vi "Property Dialog_Toggle RW Symbol.vi"(5 "Prior Property Array":T1(array[cluster]), 6 "Shift click?":bool, 7 "Action":T2, 8 "Error In":errorcluster, 9 "Coords":cluster{"Horizontal":i32, "Vertical":i32}, 10 "Tree Control in":refnum<vi>, 11 "All Tree Refs":refnum<vi>[](array[refnum])) -> (0 "Error Out":errorcluster, 1 "Tag Selected":string[](array[string]), 2 "Tree Control Out":refnum<vi>)   [LabVIEW 2023]
uses:
  controls/action enum.ctl
panel:
  out "subarray":string[](array[string])
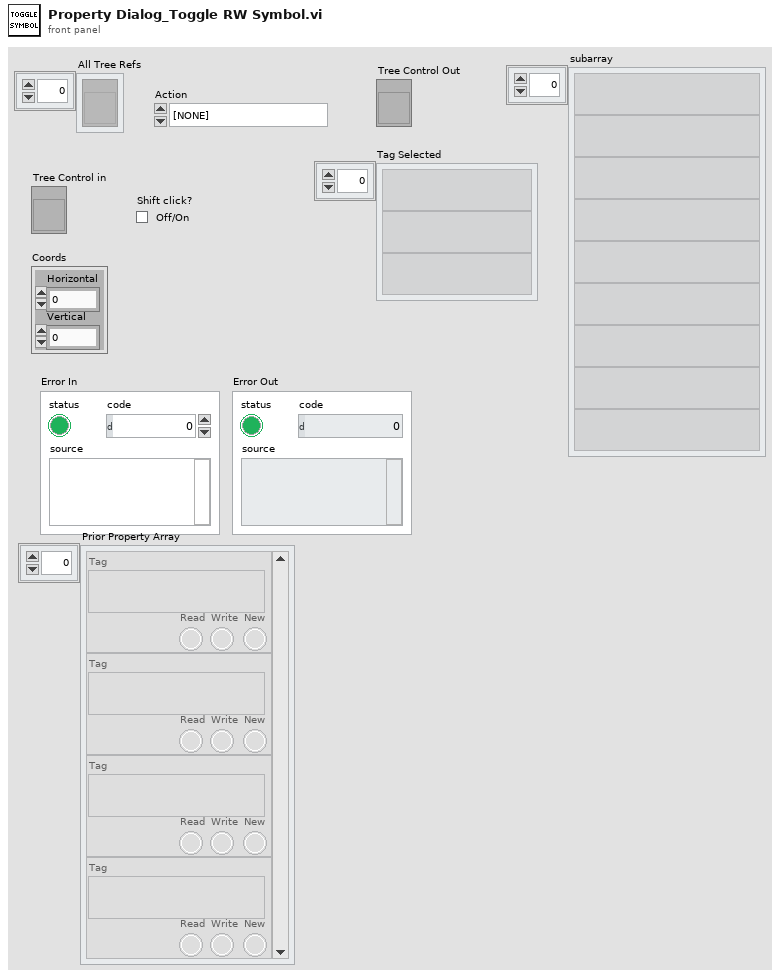
[diagram p1: front panel]
types:
  T1 = cluster{"Tag":string, "Read":bool, "Write":bool, "New":bool}[]
  T2 = typedef "action enum.ctl" = enum16{"[NONE]", "Wire Bundle", "Wire Unbundle", "Terminal Unbundle", "Terminal Bundle", "Bundler Move Up", "Bundler Move Down", "Bundler Insert", "Bundler Remove", "Bundler Remove Unwired", "Bundler Rearrange", "In Place Insert", "In Place Remove", "In Place Remove Unwired", "In Place Rearrange", "Wire Properties", "Wire Method", "Terminal Properties", "Terminal Method", "Property Move Up", "Property Move Down", "Properties Insert", "Properties Remove", "Properties Remove Unwired", "Properties Rearrange", "Method Change", "Class for Constant", "Class For Control", "Class For Node", "Class Name to Clipboard"}
  T3 = enum16{"Init", "Read", "Remove", "Remove or Append", "Append", "Append If New"}
  T4 = cluster{"Tag":string, "Read":bool, "Write":bool, "New":bool}
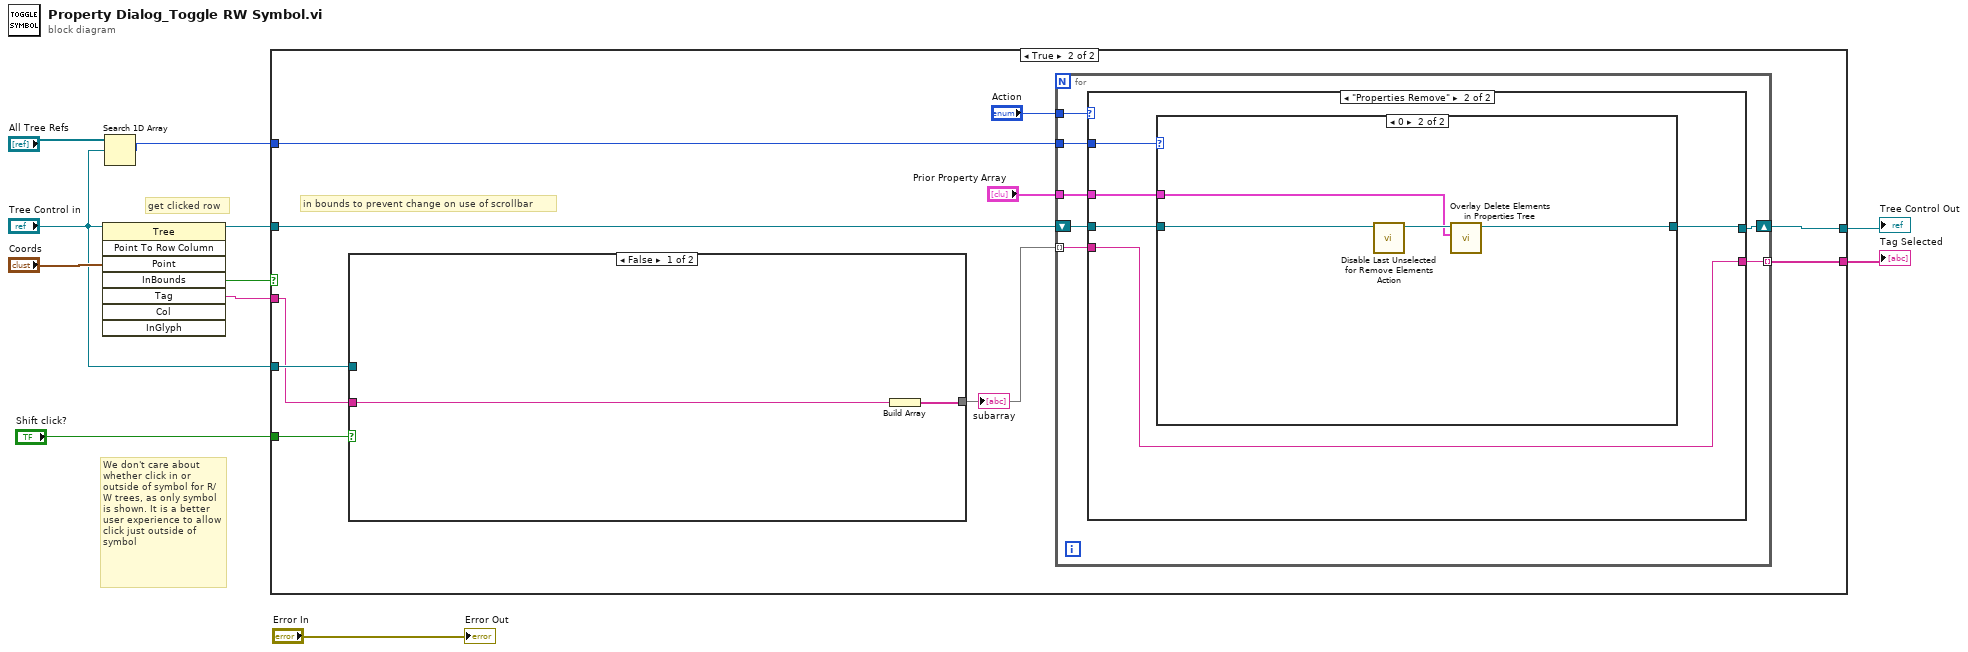
[diagram p0: block diagram]
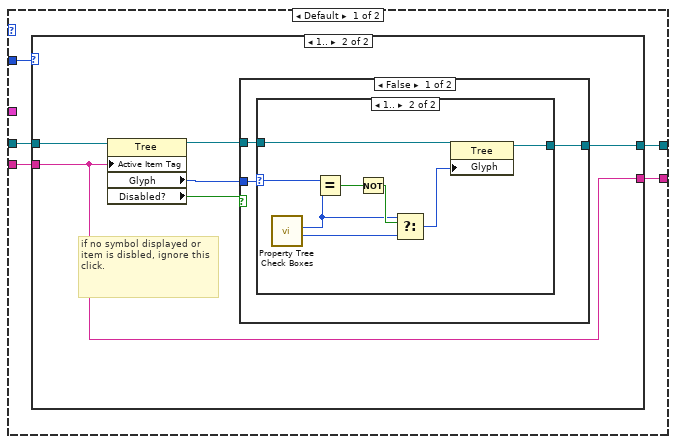
[diagram p3: hidden frame]
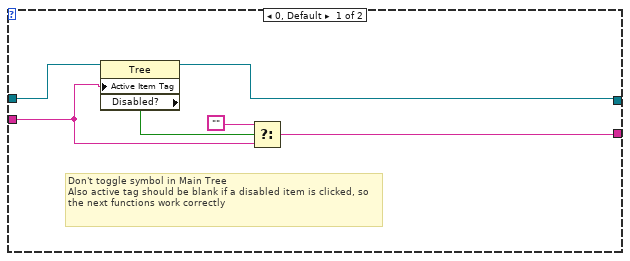
[diagram p4: hidden frame]
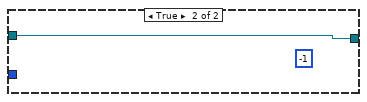
[diagram p6: hidden frame]
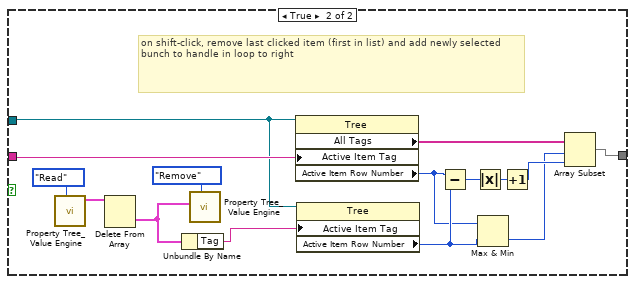
[diagram p8: hidden frame]
diagram:
  # "We don't care about whether click in or outside of symbol for R/W trees, as only symbol is shown. It is a better user experience to allow click just outside of symbol"
  # "get clicked row"
  n1 = invoke class="Tree" method="Point To Row Column"(reference="Tree Control in", "Point"="Coords") -> (reference out=w10:refnum<vi>, "InBounds"=w2:bool, "Tag"=w5:string)  [unwired: 6 in, 5 out]
  n2 = Search 1D Array(1D array="All Tree Refs", element="Tree Control in") -> (index of element=w8:i32)  [unwired: 1 in]
  n3 = case shown="True" w2 {
    tunnel: w10 -> [_ w21]
    tunnel: w8 -> [_ w20]
    tunnel: "Shift click?" -> [_ w18]
    tunnel: "Tree Control in" -> [_ w17]
    tunnel: w5 -> [_ w16]
    tunnel: [_ w14] -> w4
    tunnel: [_ w13] -> w3
    frame False {
    }
    frame True {
      # "in bounds to prevent change on use of scrollbar"
      n4 = case shown="False" w18 {
        tunnel: w17 -> [_ w73]
        tunnel: w16 -> [w70 w75]
        tunnel: [w69 w74] -> w15
        frame False {
          n5 = Build Array(w70) -> (w69:string[])
        }
        frame True {
          # "on shift-click, remove last clicked item (first in list) and add newly selected bunch to handle in loop to right"
          n6 = call "Property Tree_Value Engine.vi"("Save Action"=T3."Read" ("Action")) -> ("Property Array Out"=w85:T1)  [unwired: 8 in, 2 out]
          n7 = Delete From Array(array=w85) -> (deleted portion=w84:T4)  [unwired: 2 in, 1 out]
          n8 = Unbundle By Name(w84) -> ("Tag"=w76:string)
          n9 = call "Property Tree_Value Engine.vi"("Save Action"=T3."Remove" ("Action"), "Element"=w84) -> ()  [unwired: 7 in, 3 out]
          n10 = property class="Tree"(reference=w73, "Active Item Tag"=w75) -> ("All Tags"=w78:string[], "Active Item Row Number"=w79:i32)  [unwired: 1 in, 2 out]
          n11 = property class="Tree"(reference=w73, "Active Item Tag"=w76) -> ("Active Item Row Number"=w80:i32)  [unwired: 1 in, 2 out]
          n12 = Subtract(x=w79, y=w80) -> (x-y=w77:i32)
          n13 = Absolute Value(x=w77) -> (abs(x)=w81:i32)
          n14 = Max & Min(x=w79, y=w80) -> (min(x,y)=w82:i32)  [unwired: 1 out]
          n15 = Increment(x=w81) -> (x+1=w83:i32)
          n16 = Array Subset(array=w78, index=w82, length=w83) -> (w74:string[])
        }
      }
      "subarray" <- w15
      n17 = for {
        tunnel: w20 -> [w26]
        tunnel: "Action" -> [w25]
        shift-right: [w27] -> w13
        shift-left: w21 -> [w28]
        tunnel: w15 -> [w24] mode=indexing
        tunnel: [w23] -> w14 mode=indexing
        tunnel: "Prior Property Array" -> [w22]
        n18 = case shown="\"Properties Remove\"" w25 {
          tunnel: w28 -> [w33 w62]
          tunnel: [w32 w63] -> w27
          tunnel: w26 -> [w31 w61]
          tunnel: w24 -> [w30 w60]
          tunnel: [w29 w60] -> w23
          tunnel: w22 -> [_ w59]
          frame Default {
            n19 = case shown="1.." w31 {
              tunnel: w33 -> [w39 w45]
              tunnel: [w37 w44] -> w32
              tunnel: w30 -> [w36 w43]
              tunnel: [w34 w43] -> w29
              frame 0, Default {
                # "Don't toggle symbol in Main Tree\nAlso active tag should be blank if a disabled item is clicked, so the next functions work correctly"
                n20 = property class="Tree"(reference=w39, "Active Item Tag"=w36) -> (reference out=w37:refnum<vi>, "Disabled?"=w38:bool)  [unwired: 1 in, 1 out]
                n21 = Select(t="", s=w38, f=w36) -> (s? t:f=w34:string)
              }
              frame 1.. {
                # "if no symbol displayed or item is disbled, ignore this click."
                n22 = property class="Tree"(reference=w45, "Active Item Tag"=w43) -> (reference out=w42:refnum<vi>, "Glyph"=w41:i32, "Disabled?"=w40:bool)  [unwired: 1 in, 1 out]
                n23 = case shown="False" w40 {
                  tunnel: w42 -> [w48 w58]
                  tunnel: w41 -> [w47 _]
                  tunnel: [w46 w58] -> w44
                  frame False {
                    n24 = case shown="1.." w47 {
                      selector: w47 -> [_ w55]
                      tunnel: w48 -> [w49 w56]
                      tunnel: [w49 w52] -> w46
                      frame 0, Default {
                      }
                      frame 1.. {
                        n25 = call "Property Tree Check Boxes.vi"() -> ("Checked"=w50:i32, "Unchecked"=w51:i32)  [unwired: 9 in, 1 out]
                        n26 = Equal?(x=w55, y=w51) -> (x = y?=w54:bool)
                        n27 = Not(x=w54) -> (.not. x?=w53:bool)
                        n28 = Select(t=w51, s=w53, f=w50) -> (s? t:f=w57:i32)
                        n29 = property class="Tree"(reference=w56, "Glyph"=w57) -> (reference out=w52:refnum<vi>)  [unwired: 1 in, 1 out]
                      }
                    }
                  }
                  frame True {
                    (unwired) -1
                  }
                }
              }
            }
          }
          frame "Properties Remove" {
            n30 = case shown="0" w61 {
              tunnel: [w64 w68] -> w63
              tunnel: w62 -> [w64 w66]
              tunnel: w59 -> [_ w65]
              frame 1.., Default {
                # "Don't toggle RW symbols on remove actions."
              }
              frame 0 {
                n31 = call "Disable Last Unselected for Remove Elements Action.vi"("Tree Ref"=w66) -> ("Tree Ref Out"=w67:refnum<vi>)  [unwired: 8 in, 2 out]
                n32 = call "Overlay Delete Elements in Properties Tree.vi"("Prior Property Array"=w65, "Tree Ref"=w67) -> ("Tree Ref Out"=w68:refnum<vi>)  [unwired: 8 in, 1 out]
              }
            }
          }
        }
      }
    }
  }
  "Tree Control Out" <- w3
  "Tag Selected" <- w4
  "Error Out" <- "Error In"
